vi "getComputedParameters.vi"(0 "Microscope in":refnum<class "Microscope.lvclass">, 11 "error in (no error)":errorcluster) -> (4 "Microscope out":refnum<class "Microscope.lvclass">, 8 "Computed Parameters":T1 {"Detector Read rate" format="%#_4f"; "Actual samples to Read per Line" format="%#_4f"; "Trash Samples" format="%#_4f"; "Samples to Average" format="%#_4f"; "total pixels per line" format="%#_4f"; "Galvo Timebase divisor" format="%#_4f"; "Galvo Write rate" format="%#_4f"; "Lines/sec" format="%#_4f"; "Flyback Pixels" format="%#_4f"; "Fill Factor" format="%#_4f"; "Pixel Dwell Time (us)" format="%#_4f"; "Pixels/sec" format="%#_4f"}, 10 "Scanning Parameters":T2, 15 "error out":errorcluster)   [LabVIEW 2012, in "Microscope.lvclass"]
uses:
  classes/Microscope.lvclass
  typedefs/SyncAlgo.ctl
  classes/Microscope.lvclass/Microscope.ctl
panel:
  in  "Scanning Parameters Template":T2
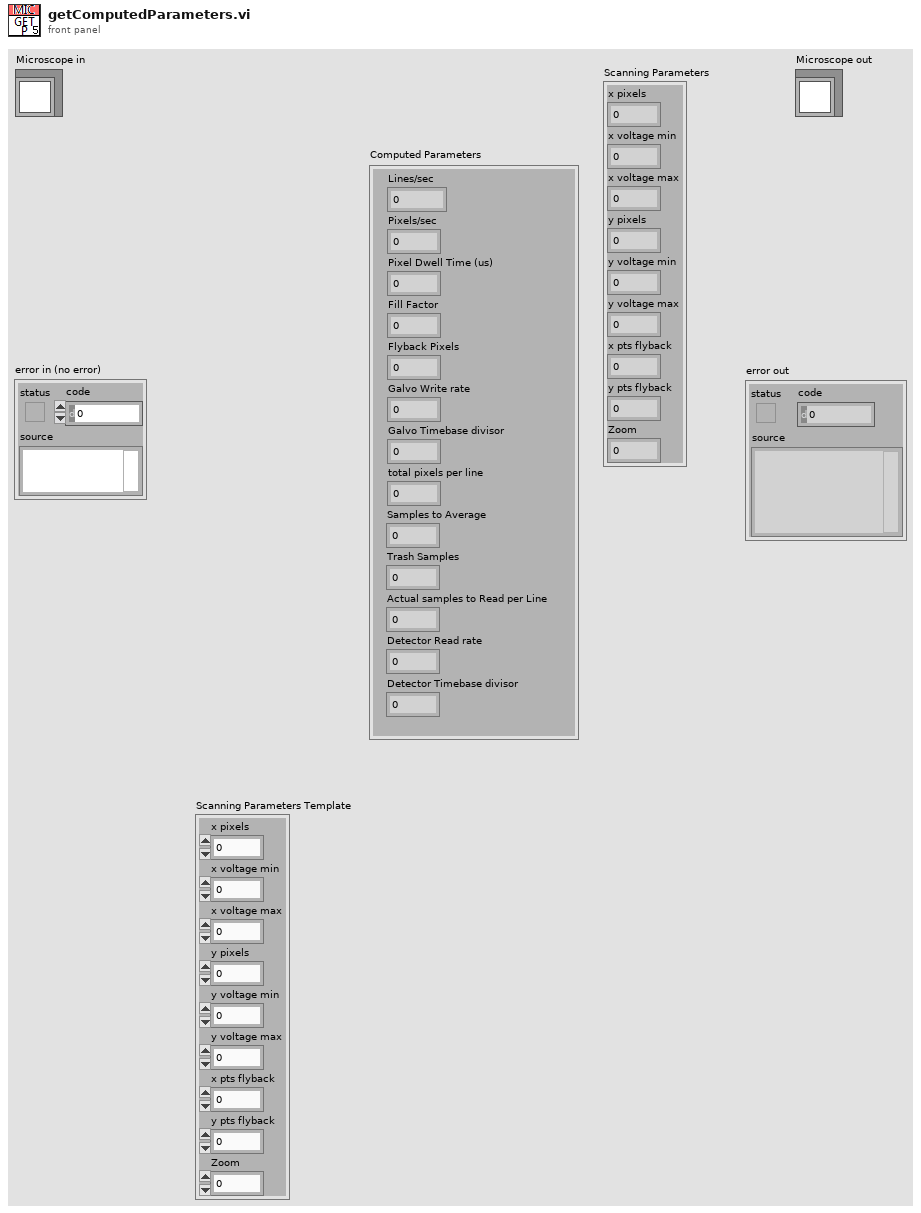
[diagram p1: front panel]
types:
  T1 = typedef "SyncAlgo.ctl" = cluster{"Pixels/sec":dbl, "Pixel Dwell Time (us)":dbl, "Fill Factor":dbl, "Flyback Pixels":dbl, "Lines/sec":dbl, "Galvo Write rate":dbl, "Galvo Timebase divisor":i32, "total pixels per line":dbl, "Samples to Average":dbl, "Trash Samples":dbl, "Actual samples to Read per Line":dbl, "Detector Read rate":dbl, "Detector Timebase divisor":i32}
  T2 = cluster{"x pixels":i32, "x voltage min":dbl, "x voltage max":dbl, "y pixels":i32, "y voltage min":dbl, "y voltage max":dbl, "x pts flyback":i32, "y pts flyback":i32, "Zoom":dbl}
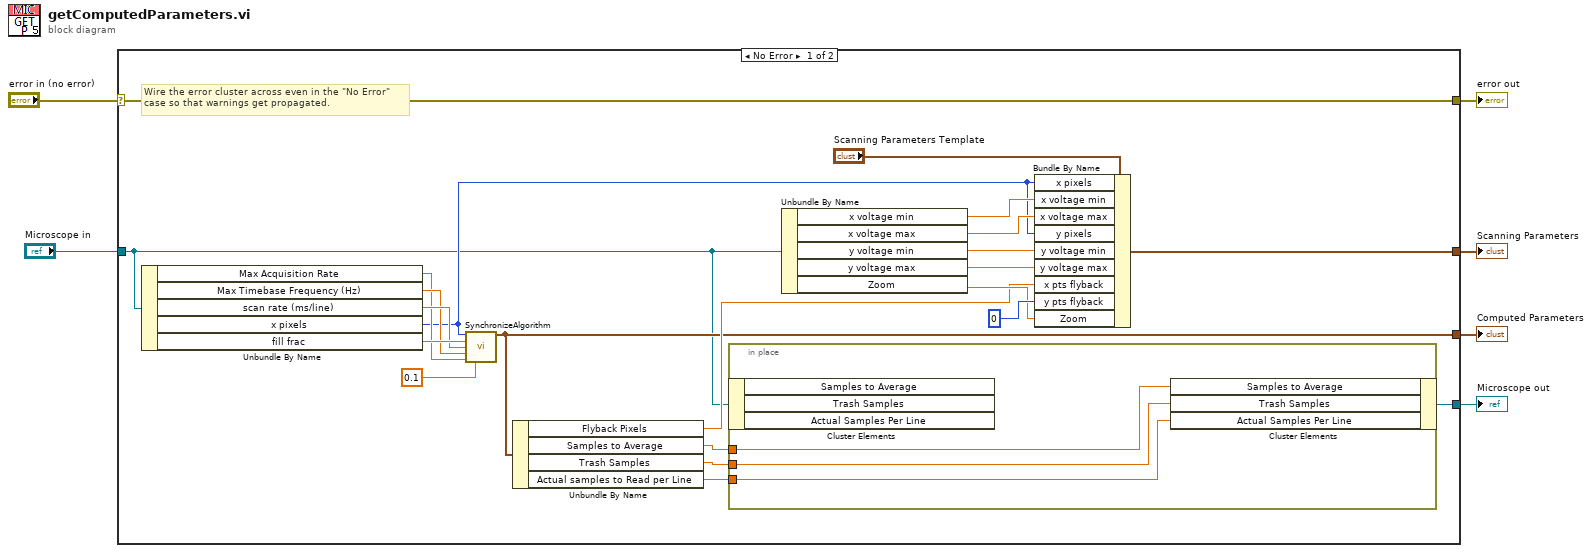
[diagram p0: block diagram]
diagram:
  n1 = case shown="No Error" "error in (no error)" {
    selector: "error in (no error)" -> [w28 w33]
    tunnel: [w28 w33] -> w5
    tunnel: [w15 w32] -> w3
    tunnel: "Microscope in" -> [w10 w32]
    tunnel: [w17 _] -> w2
    tunnel: [w11 _] -> w1
    frame No Error {
      # "Wire the error cluster across even in the \"No Error\"\ncase so that warnings get propagated."
      n2 = Unbundle By Name(w10) -> ("Max Acquisition Rate"=w24:dbl, "Max Timebase Frequency (Hz)"=w25:dbl, "scan rate (ms/line)"=w26:dbl, "x pixels"=w12:i32, "fill frac"=w27:dbl)
      n3 = call "SynchronizeAlgorithm.vi"("xpixels"=w12, "fill factor"=w27, "ms/line"=w26, "maximum timebase frequency"=w25, "Detector maximum sampling rate"=w24, "tolerance"=0.1) -> ("Output Cluster"=w11:T1)  [unwired: 8 in, 1 out]
      n4 = Unbundle By Name(w11) -> ("Flyback Pixels"=w13:dbl, "Samples to Average"=w9:dbl, "Trash Samples"=w8:dbl, "Actual samples to Read per Line"=w7:dbl)
      n5 = in-place {
        in-place-border: w9 -> [w30]
        in-place-border: w8 -> [w31]
        in-place-border: w7 -> [w29]
        n6 = in-place-cluster #1(w10) -> ()  [unwired: 3 out]
        n7 = in-place-cluster #1("Samples to Average"=w30, "Trash Samples"=w31, "Actual Samples Per Line"=w29) -> (w15:refnum<class "Microscope.lvclass">)
      }
      n8 = Unbundle By Name(w10) -> ("x voltage min"=w23:dbl, "x voltage max"=w22:dbl, "y voltage min"=w21:dbl, "y voltage max"=w20:dbl, "Zoom"=w18:dbl)
      n9 = Bundle By Name(cluster="Scanning Parameters Template", "x pixels"=w12, "x voltage min"=w23, "x voltage max"=w22, "y pixels"=w12, "y voltage min"=w21, "y voltage max"=w20, "x pts flyback"=w13, "y pts flyback"=0, "Zoom"=w18) -> (w17:T2)
    }
    frame Error {
    }
  }
  "error out" <- w5
  "Microscope out" <- w3
  "Scanning Parameters" <- w2
  "Computed Parameters" <- w1
